vi "Read Encoder Data.vi"(8 "error in":errorcluster, 11 "FPGA VI Reference In":refnum<k20>) -> (0 "error out":errorcluster, 2 "Array":dbl[](array[numeric]), 3 "FPGA VI Reference Out":refnum<k20>)   [LabVIEW 2009]
uses:
  <vilib>/rvi/interface/nirviReadWriteControl/nirviReadWriteControl.xnode
  FPGA Bitfiles/sbRIOController.lv~4B_sbRIO-9642_FPGA Main NoStartE~C3.lvbitx
  FPGA/FPGA Main NoStartEnc.vi
  <vilib>/Utility/error.llb/Error Cluster From Error Code.vi
  <vilib>/rvi/errors/niLvFpgaAdjustHostInterfaceError.vi
  <vilib>/rvi/interface/common/niFpgaNodeNameForErrorReporting.ctl
  <vilib>/rvi/errors/niLvFpgaWhatHappensToTopLevelVI.ctl
  NiRioSrv.dll
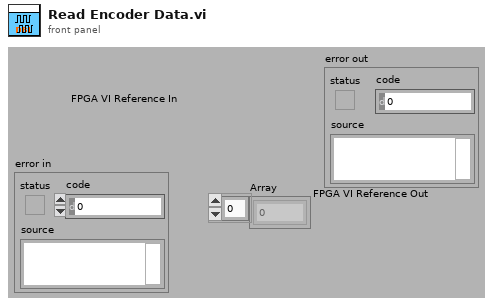
[diagram p1: front panel]
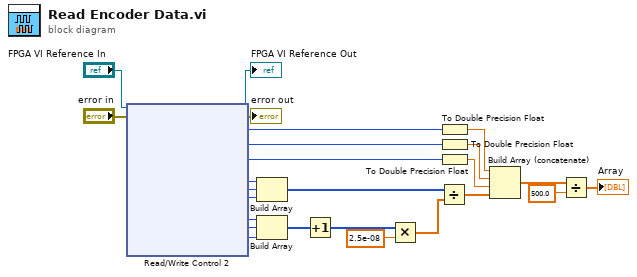
[diagram p0: block diagram]
diagram:
  n1 = xnode ("Read/Write Control 2")("FPGA VI Reference In"="FPGA VI Reference In", "error in"="error in") -> ("FPGA VI Reference Out"=→"FPGA VI Reference Out":refnum<k20>, "error out"=→"error out":errorcluster, "Elevation Position"=w5:i32, "Pitch Position"=w14:i32, "Travel Position"=w13:i32, "Elevation Velocity"=w21:i32, "Pitch Velocity"=w22:i32, "Travel Velocity"=w23:i32, "Elevation dT (Ticks)"=w15:u32, "Pitch dT (Ticks)"=w16:u32, "Travel dT (Ticks)"=w17:u32)
  n2 = Build Array(w21, w22, w23) -> (w24:i32[])
  n3 = Build Array(w15, w16, w17) -> (w18:u32[])
  n4 = Increment(x=w18) -> (x+1=w3:u32[])
  n5 = Multiply(x=w3, y=2.5e-08) -> (x*y=w20:dbl[])
  n6 = Divide(x=w24, y=w20) -> (x/y=w25:dbl[])
  n7 = To Double Precision Float(number=w5) -> (double precision float=w12:dbl)
  n8 = To Double Precision Float(number=w14) -> (double precision float=w11:dbl)
  n9 = To Double Precision Float(number=w13) -> (double precision float=w10:dbl)
  n10 = Build Array (concatenate)(w12, w11, w10, w25) -> (w4:dbl[])
  n11 = Divide(x=w4, y=500.0) -> (x/y=→"Array":dbl[])
